vi "addError.vi"(7 "execution time (sec)":dbl, 8 "error in (no error)":errorcluster, 9 "test error":errorcluster, 10 "test":refnum<class>, 11 "TestTestResult in":refnum<class "_TextTestResult.lvclass">) -> (0 "error out":errorcluster, 3 "TestTestResult out":refnum<class "_TextTestResult.lvclass">)   [LabVIEW 2013, in "_TextTestResult.lvclass"]
uses:
  _TextTestResult.lvclass
  TestCase/TestCase.lvclass
  TestResult/TestResult.lvclass
  _TextTestResult.lvclass/_TextTestResult.ctl
panel:
  # "JKI VI Tester for LabVIEW\nhttp://jkisoft.com/vi-tester\nCopyright (C) 2007-2009, JKI <info@jkisoft.com>\nALL RIGHTS RESERVED"
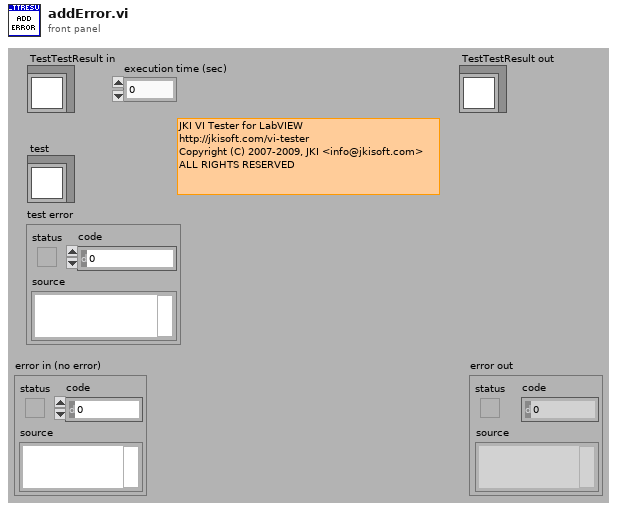
[diagram p1: front panel]
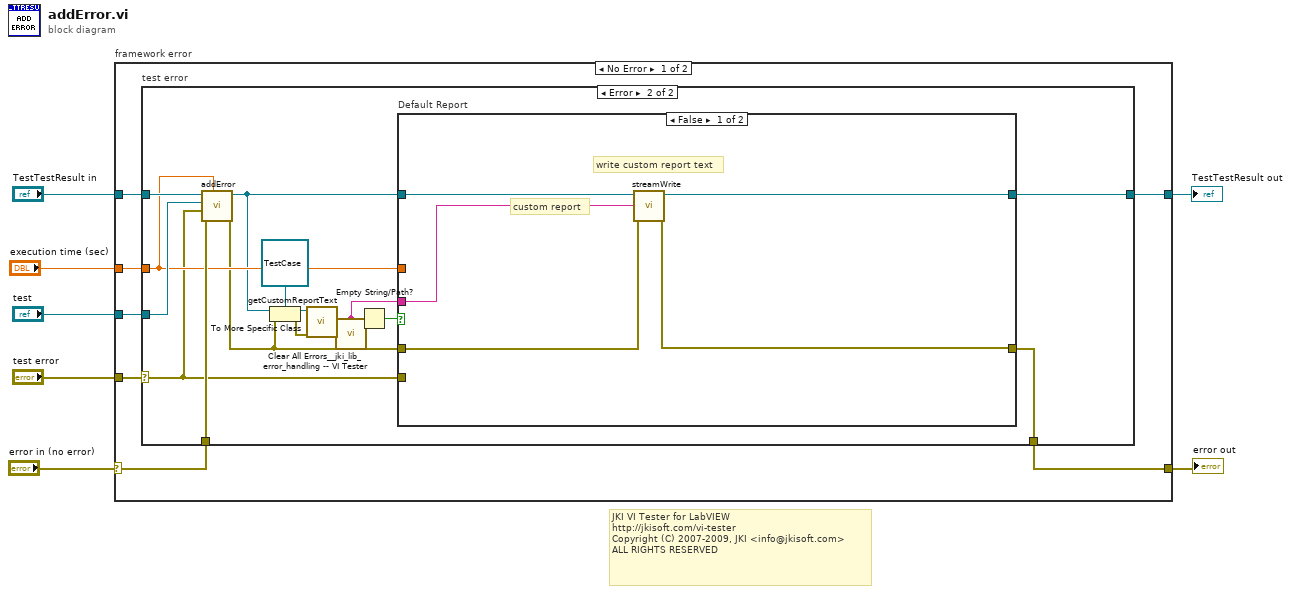
[diagram p0: block diagram]
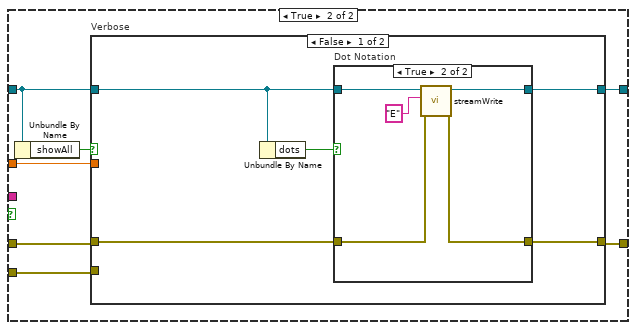
[diagram p3: hidden frame]
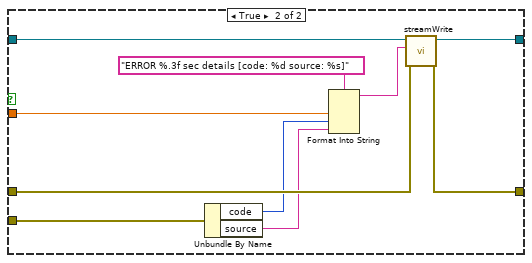
[diagram p5: hidden frame]
diagram:
  # "JKI VI Tester for LabVIEW\nhttp://jkisoft.com/vi-tester\nCopyright (C) 2007-2009, JKI <info@jkisoft.com>\nALL RIGHTS RESERVED"
  n1 = case "framework error" shown="No Error" "error in (no error)" {
    selector: "error in (no error)" -> [w12 w67]
    tunnel: [w10 w67] -> w6
    tunnel: [w11 w66] -> w4
    tunnel: "TestTestResult in" -> [w14 w66]
    tunnel: "test error" -> [w9 _]
    tunnel: "test" -> [w13 _]
    tunnel: "execution time (sec)" -> [w8 _]
    frame No Error {
      n2 = case "test error" shown="Error" w9 {
        selector: w9 -> [_ w25]
        tunnel: w14 -> [w16 w31]
        tunnel: w13 -> [_ w30]
        tunnel: w12 -> [w15 w29]
        tunnel: [w16 w28] -> w11
        tunnel: [w15 w27] -> w10
        tunnel: w8 -> [_ w26]
        frame No Error {
        }
        frame Error {
          n3 = call-parent "addError.vi"("execution time (sec)"=w26, "error in (no error)"=w29, "test error"=w25, "test"=w30, "TestResult in"=w31) -> ("error out"=w19:errorcluster, "TestResult out"=w20:refnum<class "_TextTestResult.lvclass">)  [unwired: 5 in]
          n4 = To More Specific Class(target class=refnum<class "TestCase.lvclass"> refnum ("TestCase in"), reference=w20, error in=w19) -> (specific class reference=w22:refnum<class "TestCase.lvclass">, error out=w24:errorcluster)
          n5 = call-dynamic "getCustomReportText.vi"("error in (no error)"=w24, "TestCase in"=w22) -> ("error out"=w21:errorcluster, "customReportText"=w17:string)  [unwired: 7 in, 1 out]
          n6 = call "Clear All Errors__jki_lib_error_handling -- VI Tester.vi"("error in"=w21) -> ()  [unwired: 4 in, 1 out]
          n7 = Empty String/Path?(string/path=w17) -> (empty?=w18:bool)
          n8 = case "Default Report" shown="False" w18 {
            tunnel: [w35 w42] -> w28
            tunnel: [w33 w41] -> w27
            tunnel: w26 -> [_ w40]
            tunnel: w25 -> [_ w39]
            tunnel: w20 -> [w36 w38]
            tunnel: w19 -> [w34 w37]
            tunnel: w17 -> [w32 _]
            frame False {
              # "custom report"
              # "write custom report text"
              n9 = call "streamWrite.vi"("error in (no error)"=w34, "String"=w32, "TestTestResult in"=w36) -> ("error out"=w33:errorcluster, "TestTestResult out"=w35:refnum<class "_TextTestResult.lvclass">)  [unwired: 7 in]
            }
            frame True {
              n10 = Unbundle By Name(w38) -> ("showAll"=w43:bool)
              n11 = case "Verbose" shown="False" w43 {
                tunnel: w38 -> [w47 w65]
                tunnel: w37 -> [w45 w63]
                tunnel: [w44 w62] -> w41
                tunnel: [w48 w64] -> w42
                tunnel: w40 -> [_ w59]
                tunnel: w39 -> [_ w58]
                frame False {
                  n12 = Unbundle By Name(w47) -> ("dots"=w46:bool)
                  n13 = case "Dot Notation" shown="True" w46 {
                    tunnel: w47 -> [w49 w55]
                    tunnel: w45 -> [w50 w52]
                    tunnel: [w50 w51] -> w44
                    tunnel: [w49 w54] -> w48
                    frame False {
                    }
                    frame True {
                      n14 = call "streamWrite.vi"("error in (no error)"=w52, "String"="E" ("element"), "TestTestResult in"=w55) -> ("error out"=w51:errorcluster, "TestTestResult out"=w54:refnum<class "_TextTestResult.lvclass">)  [unwired: 7 in]
                    }
                  }
                }
                frame True {
                  n15 = Unbundle By Name(w58) -> ("code"=w57:i32, "source"=w56:string)
                  n16 = Format Into String(format string="ERROR %.3f sec details [code: %d source: %s]" ("element"), w59, w57, w56) -> (resulting string=w60:string)  [unwired: 2 in, 1 out]
                  n17 = call "streamWrite.vi"("error in (no error)"=w63, "String"=w60, "TestTestResult in"=w65) -> ("error out"=w62:errorcluster, "TestTestResult out"=w64:refnum<class "_TextTestResult.lvclass">)  [unwired: 7 in]
                }
              }
            }
          }
        }
      }
    }
    frame Error {
    }
  }
  "error out" <- w6
  "TestTestResult out" <- w4
